vi "Get Diagram Constant refs.vi"(11 "Diagram ref.":refnum<vi>) -> (1 "StringConstant refs[]":refnum<vi>[](array[refnum]), 2 "DigitalNumericConstant refs[]":refnum<vi>[](array[refnum]), 3 "alltop objects refs[]":string[](array[string]))   [LabVIEW 2014]
doc: "Returns Constant ownes by Diagram. So if you put numeric constants or string constants or now somewhere on diagram and they are not bounded any structure like WhileLoop or ForLoop, this function returns their references.\n\nFor now returns just DigitalNumericConstant and StringConstant refs as arrays."
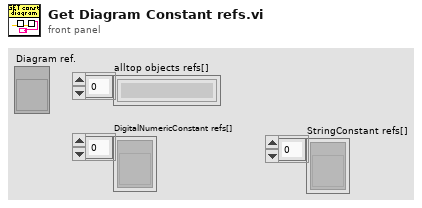
[diagram p1: front panel]
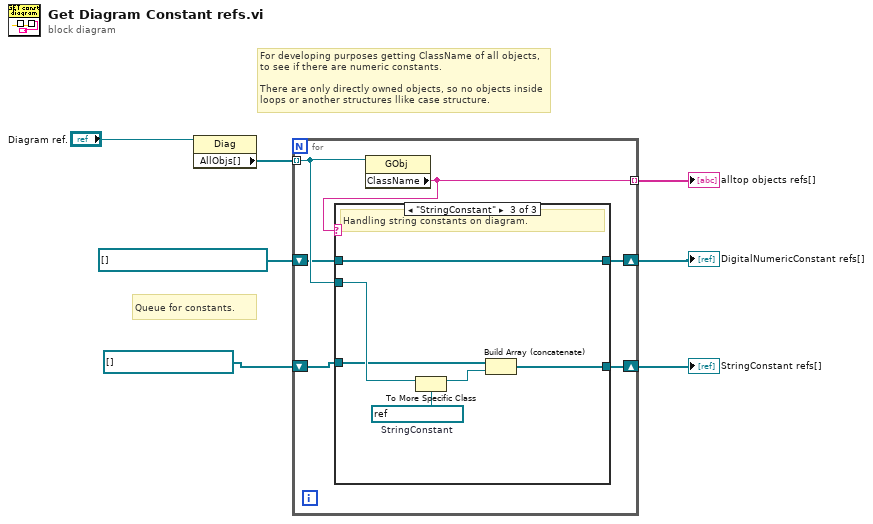
[diagram p0: block diagram]
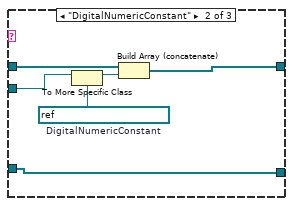
[diagram p3: hidden frame]
diagram:
  # "Queue for constants."
  # "For developing purposes getting ClassName of all objects, to see if there are numeric constants.\n\nThere are only directly owned objects, so no objects inside loops or another structures llike case structure."
  n1 = property on="Property Node" class="Diag"(reference="Diagram ref.") -> ("AllObjs[]"=w4:refnum<vi>[])  [unwired: 1 in, 2 out]
  n2 = for {
    tunnel: w4 -> [w12] mode=indexing
    tunnel: [w13] -> w5 mode=indexing
    shift-right: [w11] -> w7
    shift-left: refnum<vi>[] [] -> [w10]
    shift-right: [w8] -> w1
    shift-left: refnum<vi>[] [] -> [w9]
    n3 = property class="GObj"(reference=w12) -> ("ClassName"=w13:string)  [unwired: 1 in, 2 out]
    n4 = case shown="\"StringConstant\"" w13 {
      tunnel: w12 -> [_ w18 w26]
      tunnel: [w15 w21 w22] -> w11
      tunnel: w10 -> [w15 w20 w22]
      tunnel: w9 -> [w14 w16 w24]
      tunnel: [w14 w16 w23] -> w8
      frame Default {
      }
      frame "DigitalNumericConstant" {
        w19 = refnum<vi> refnum  # DigitalNumericConstant
        n5 = To More Specific Class(target class=w19, reference=w18) -> (specific class reference=w17:refnum<vi>)  [unwired: 1 in, 1 out]
        n6 = Build Array (concatenate)(w20, w17) -> (w21:refnum<vi>[])
      }
      frame "StringConstant" {
        w27 = refnum<vi> refnum  # StringConstant
        # "Handling string constants on diagram."
        n7 = To More Specific Class(target class=w27, reference=w26) -> (specific class reference=w25:refnum<vi>)  [unwired: 1 in, 1 out]
        n8 = Build Array (concatenate)(w24, w25) -> (w23:refnum<vi>[])
      }
    }
  }
  "DigitalNumericConstant refs[]" <- w7
  "alltop objects refs[]" <- w5
  "StringConstant refs[]" <- w1
